vi "svc_Exponential Average (1 Ch) (SGL).vi"(10 "normalized time constant (0 = use array length)":sgl, 11 "x":sgl[](array[numeric])) -> (3 "exponential average":sgl=nan)   [LabVIEW 2017]
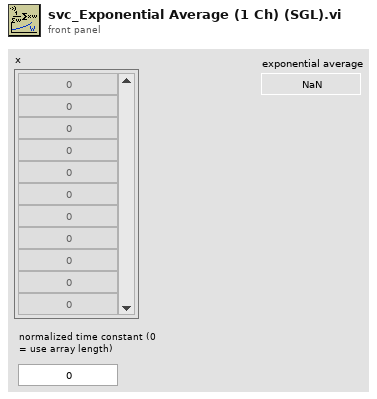
[diagram p1: front panel]
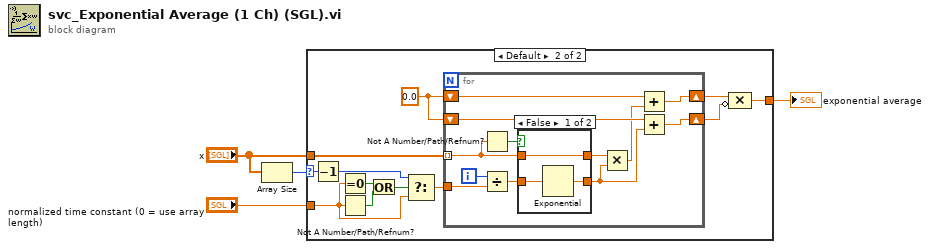
[diagram p0: block diagram]
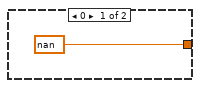
[diagram p2: hidden frame]
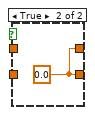
[diagram p3: hidden frame]
diagram:
  n1 = Array Size(array="x") -> (size(s)=w1:i32)
  n2 = case shown="Default" w1 {
    selector: w1 -> [_ w10]
    tunnel: [sgl nan w14] -> w4
    tunnel: "x" -> [_ w12]
    tunnel: "normalized time constant (0 = use array length)" -> [_ w6]
    frame 0 {
    }
    frame Default {
      w17 = sgl 0.0
      n3 = Decrement(x=w10) -> (x-1=w9:i32)
      n4 = Equal To 0?(x=w6) -> (x = 0?=w13:bool)
      n5 = Not A Number/Path/Refnum?(number/path/refnum=w6) -> (NaN/Path/Refnum?=w8:bool)
      n6 = Or(x=w13, y=w8) -> (x .or. y?=w7:bool)
      n7 = Select(t=w9, s=w7, f=w6) -> (s? t:f=w11:sgl)
      n8 = for {
        tunnel: w12 -> [w18] mode=indexing
        tunnel: w11 -> [w28]
        shift-right: [w22] -> w15
        shift-left: w17 -> [w26]
        shift-right: [w24] -> w16
        shift-left: w17 -> [w25]
        i -> [w29]
        n9 = Not A Number/Path/Refnum?(number/path/refnum=w18) -> (NaN/Path/Refnum?=w20:bool)
        n10 = Divide(x=w29, y=w28) -> (x/y=w27:sgl)
        n11 = case shown="False" w20 {
          tunnel: w27 -> [w32 _]
          tunnel: [w31 w33] -> w21
          tunnel: [w30 w33] -> w19
          tunnel: w18 -> [w30 _]
          frame False {
            n12 = Exponential(1:w32) -> (0:w31:sgl)
          }
          frame True {
            w33 = sgl 0.0
          }
        }
        n13 = Multiply(x=w19, y=w21) -> (x*y=w23:sgl)
        n14 = Add(x=w26, y=w23) -> (x+y=w22:sgl)
        n15 = Add(x=w25, y=w21) -> (x+y=w24:sgl)
      }
      n16 = Compound Arithmetic op=MULTIPLY(w15, invert w16) -> (w14:sgl)
    }
  }
  "exponential average" <- w4
